vi "Magnetometer_Test_v0.vi"() -> ()   [LabVIEW 2019]
uses:
  <vilib>/DAQmx/write.llb/DAQmx Write (Analog DBL 1Chan 1Samp).vi
  <vilib>/DAQmx/read.llb/DAQmx Read (Analog 1D Wfm NChan NSamp).vi
  <extravilib>/ChannelInstances/Tag-c(bool,i32,str)/Read With Abort.vi
  <extravilib>/ChannelInstances/Tag-a[.](wfm(dbl))/Read With Abort.vi
  <extravilib>/ChannelInstances/Tag-bool/Read With Abort.vi
  <extravilib>/ChannelInstances/Tag-bool/Write With Abort.vi
  <extravilib>/ChannelInstances/Tag-c(bool,i32,str)/Write With Abort.vi
  <extravilib>/ChannelInstances/Tag-a[.](wfm(dbl))/Write With Abort.vi
  <vilib>/DAQmx/create/channels.llb/DAQmx Create Channel (AI-Voltage-Basic).vi
  <vilib>/DAQmx/configure/timing.llb/DAQmx Timing (Sample Clock).vi
  <vilib>/Utility/file.llb/Write Delimited Spreadsheet (string).vi
  <vilib>/DAQmx/create/channels.llb/DAQmx Create Channel (AO-Voltage-Basic).vi
  <extravilib>/ChannelInstances/Tag-bool/Instantiate.vi
  <extravilib>/ChannelInstances/Tag-bool/EndpointRead.vi
  <vilib>/DAQmx/miscellaneous.llb/DAQmx Fill In Error Info.vi
  <extravilib>/ChannelInstances/Tag-bool/Endpoint.vi
  <extravilib>/ChannelInstances/Tag-a[.](wfm(dbl))/Instantiate.vi
  <extravilib>/ChannelInstances/Tag-c(bool,i32,str)/Instantiate.vi
  <extravilib>/ChannelInstances/Tag-c(bool,i32,str)/EndpointRead.vi
  <extravilib>/ChannelInstances/Tag-a[.](wfm(dbl))/EndpointRead.vi
  <vilib>/imath/engines/lvmath2/RunTimeEngine/Managers/WorkSpace/UID Generator.vi
  <vilib>/imath/engines/lvmath2/RunTimeEngine/RunTimeType/NIMS_RunTimeType_From StrictType (excl LVString).vi
  <instcachedir>/0/NIMS_RunTimeType_From StrictType (excl LVString)_D8AFBA86A94845AAA577C895450664BD.lvgen/NIMS_RunTimeType_From StrictType (excl LVString)_D8AFBA86A94845AAA577C895450664BD_000.vi
  <vilib>/imath/engines/lvmath2/RunTimeEngine/LocalVariableDefStatement/MC_LocalVariableDefStatement_Display.vi
  <vilib>/imath/engines/lvmath2/RunTimeEngine/ArithmeticOperatorToken/NIMS_ArithmeticOperator_power(S).vi
  <instcachedir>/0/NIMS_ArithmeticOperator_power(S)_F1497A2DE3CE4E82B2C3646D59904248.lvgen/NIMS_ArithmeticOperator_power(S)_F1497A2DE3CE4E82B2C3646D59904248_010.vi
  <vilib>/imathl/engines/lvmath/Functions/Error Handling/Create Error.vi
  <vilib>/imath/engines/lvmath2/RunTimeEngine/Managers/SymbolTable/Clear UID.vi
  <vilib>/imath/engines/lvmath2/RunTimeEngine/NodeEndStatement/NIMS_NodeEndStatement_Output.vi
  <instcachedir>/0/NIMS_NodeEndStatement_Output_53EC0D466D134D7ABD903AC30B43404B.lvgen/NIMS_NodeEndStatement_Output_53EC0D466D134D7ABD903AC30B43404B_009.vi
  <vilib>/imath/engines/lvmath2/RunTimeEngine/ErrorHandling/NIMS_Finalize Error.vi
  <extravilib>/ChannelInstances/Tag-a[.](wfm(dbl))/Endpoint.vi
  <extravilib>/ChannelInstances/Tag-c(bool,i32,str)/Endpoint.vi
  <vilib>/DAQmx/write.llb/DAQmx Write (Analog 1D DBL NChan 1Samp).vi
  <resource>/objmgr/daqmx.rc
  <extravilib>/ChannelInstances/Tag-bool.lvlib
  <extravilib>/ChannelInstances/Tag-c(bool,i32,str).lvlib
  <extravilib>/ChannelInstances/Tag-a[.](wfm(dbl)).lvlib
  <vilib>/imath/engines/lvmath2/RunTimeEngine/Managers/SymbolTable/NIMS_WorkSpace.lvlib
panel:
  in  "Data Record Work Rate (ms)":u16(ring)=100 items=["100"=100, "250"=250, "500"=500, "1000"=1000, "2500"=2500, "5000"=5000, ""=0]
  out "Magnetic Field Indicator":dbl
  out "Magnetic Field":dbl(graph)
  out "Temperature (VDC)":dbl
  out "Temperature (Celsius)":dbl
  out "Temperature":dbl(slide) scale=-40.0..160.0
  in  "Temperature \nMeasurement On/Off":bool=TRUE
  out "TCP Connection":bool
  in  "Reset":bool
  out "Output 2 Current In Range?":bool
  out "Output 1 Current In Range?":bool
  out "Output 2 Input Current":string
  out "Output 1 Measured Current":string
  out "Output 2 Input Voltage":string
  out "Output 2 Measured Current":string
  out "Output 2 Measured Voltage":string
  out "Output 1 Input Current":string
  out "Output 1 Input Voltage":string
  out "Output 1 Measured Voltage":string
  in  "Output On/Off":bool
  out "Iteration of PS Controller":dbl
  out "MtM Z-Axis Output Voltage":string
  out "MtM Y-Axis Output Voltage":string
  in  "Data History Work Rate (ms)":u16(ring)=1000 items=["100"=100, "250"=250, "500"=500, "1000"=1000, "2500"=2500, "5000"=5000, ""=0]
  out "MtM X-Axis Output Voltage":string
  in  "Simulation On/Off":bool
  in  "Sample Clock Source":tag="OnboardClock"
  out "MtM Z-Axis Output Voltage":waveform(dbl)(graph)
  out "MtM Y-Axis Output Voltage":waveform(dbl)(graph)
  out "MtM X-Axis Output Voltage":waveform(dbl)(graph)
  in  "MtM Z-Axis Input Voltage":dbl
  in  "MtM Y-Axis Input Voltage":dbl
  in  "MtM X-Axis Input Voltage":dbl
  in  "Acquire Buffer Size":i32=1024
  in  "Sample Rate":dbl=1000.0 format="%0.2f"
  out "DAQmx Read Rate":dbl
  in  "Number of Samples":i32=100
  out "While loop duration (ms)":u32
  in  "Stop":bool
  # "Sensor Output"
  # "Data Acqusition Timing and\nBuffer Settings"
  # "Temperature Output"
  # "Acquire Data History"
  # "Magnetic Field Output"
  # "Power Supply Control and Status"
  # "Simulation of Analogue Voltage Generation"
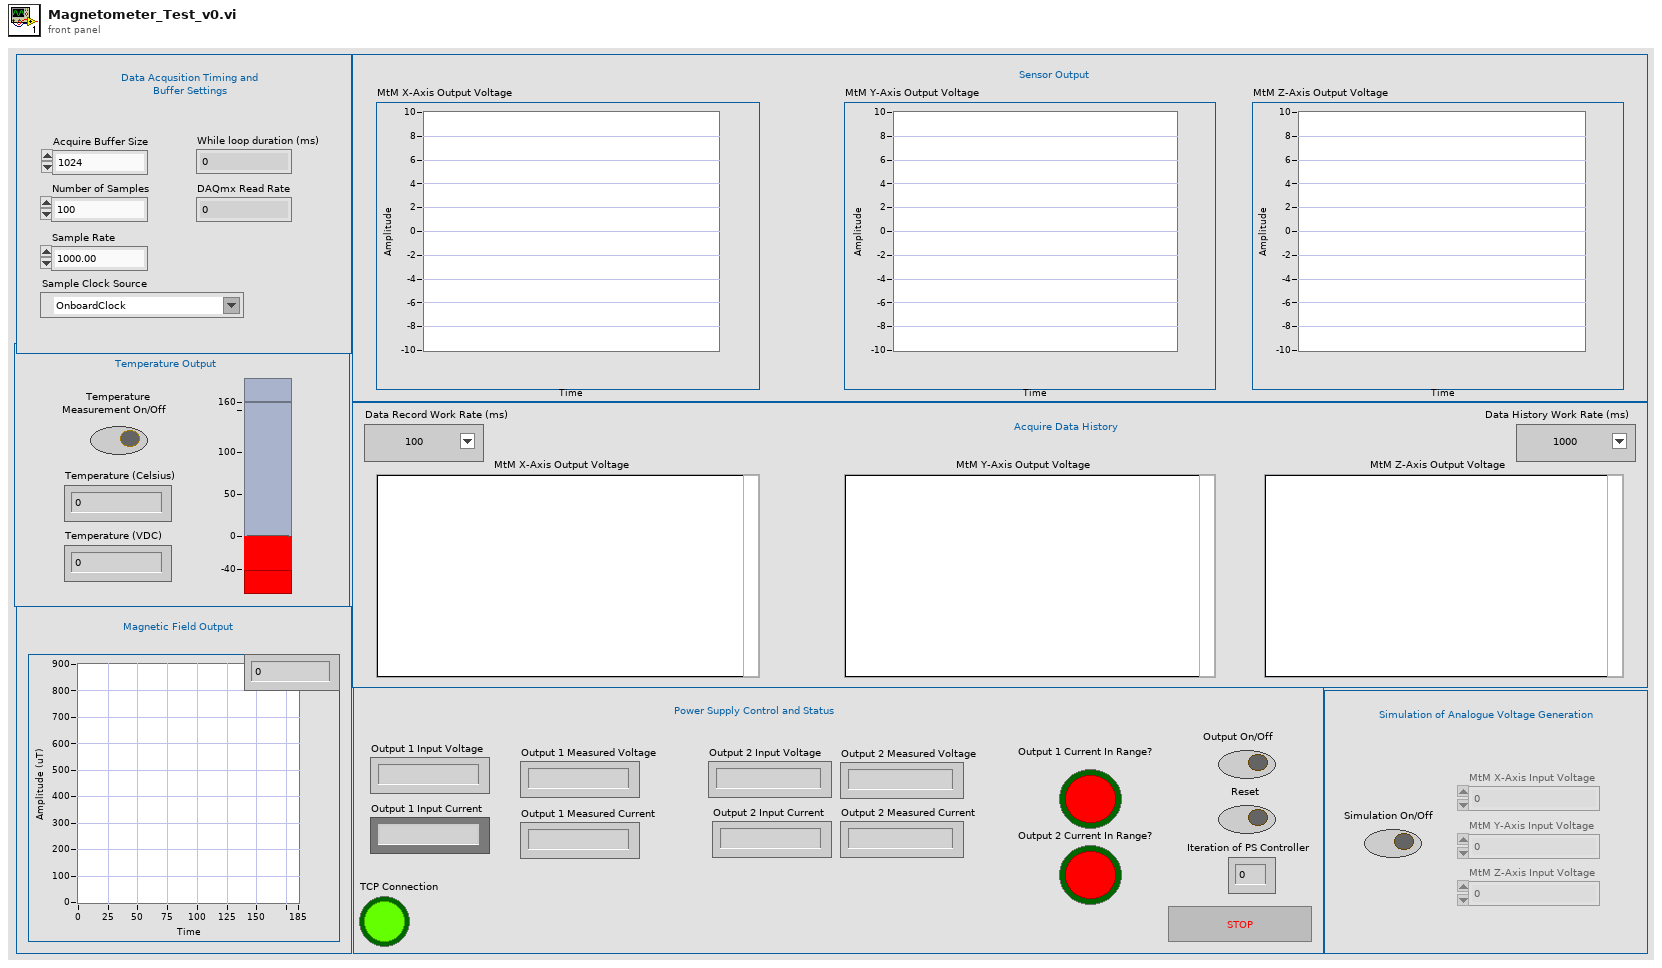
[diagram p1: front panel]
types:
  T1 = typedef "Tag-bool.lvlib/))Channel.ctl" = refnum<queue>
  T2 = typedef "Tag-a[.](wfm(dbl)).lvlib/))Channel.ctl" = refnum<queue>
  T3 = typedef "Tag-c(bool,i32,str).lvlib/))Channel.ctl" = refnum<queue>
  T4 = enum8{"Enabled", "Disabled", "Disabled and Grayed Out"}
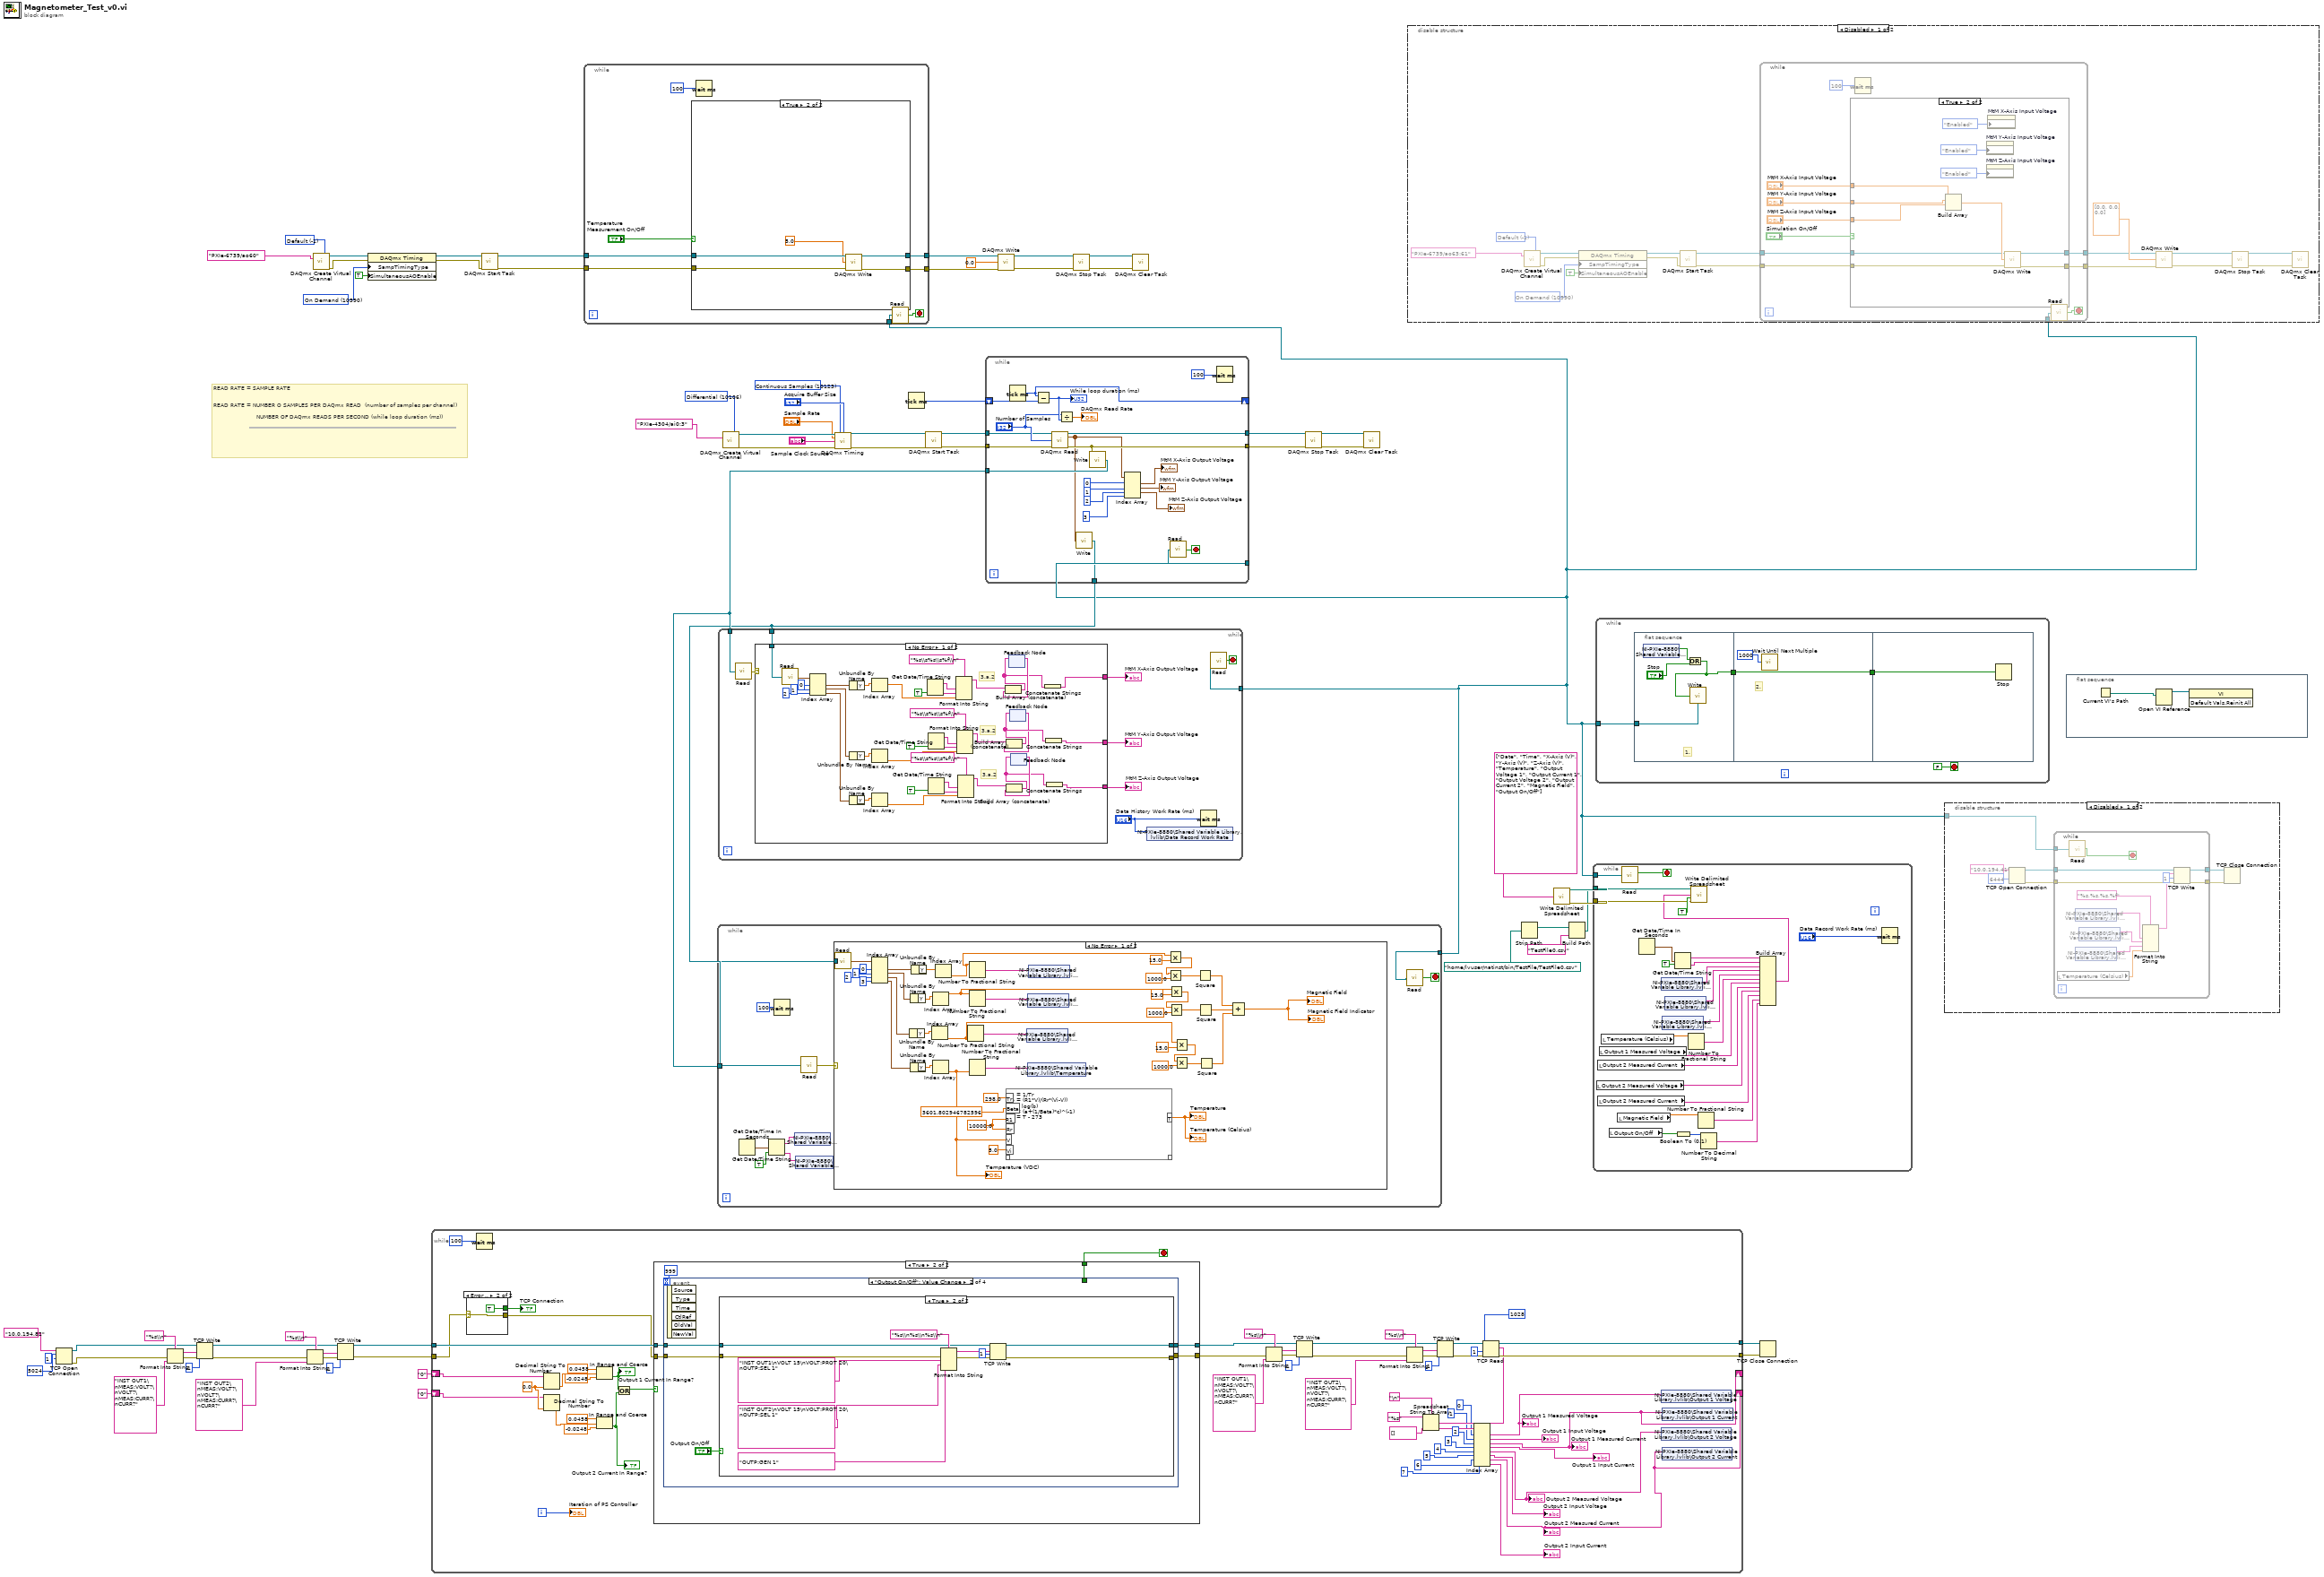
[diagram p0: block diagram]
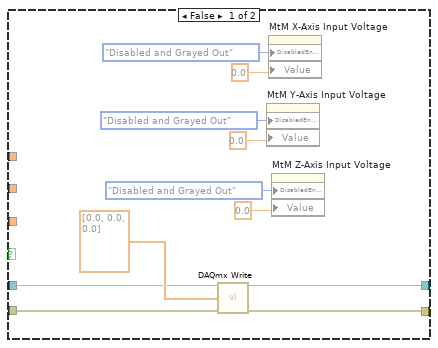
[diagram p4: hidden frame]
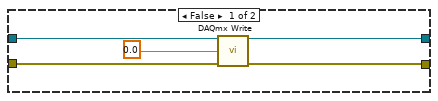
[diagram p6: hidden frame]
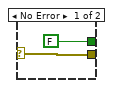
[diagram p7: hidden frame]
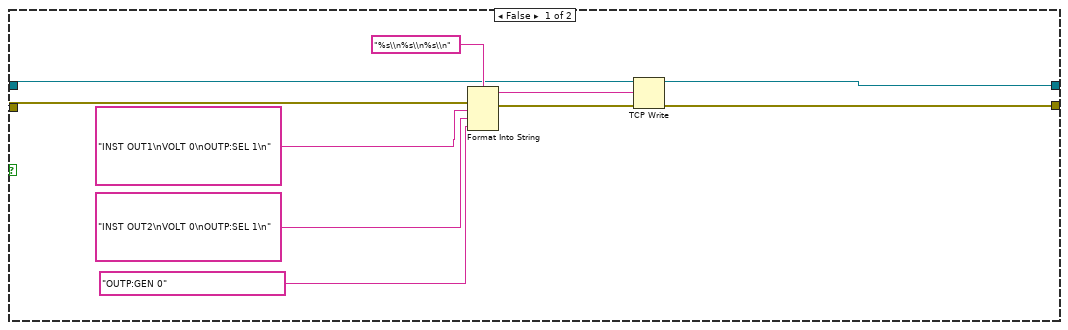
[diagram p8: hidden frame]
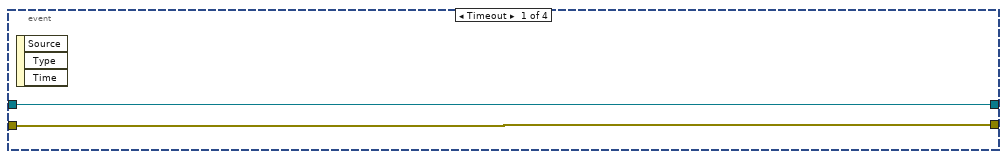
[diagram p9: hidden frame]
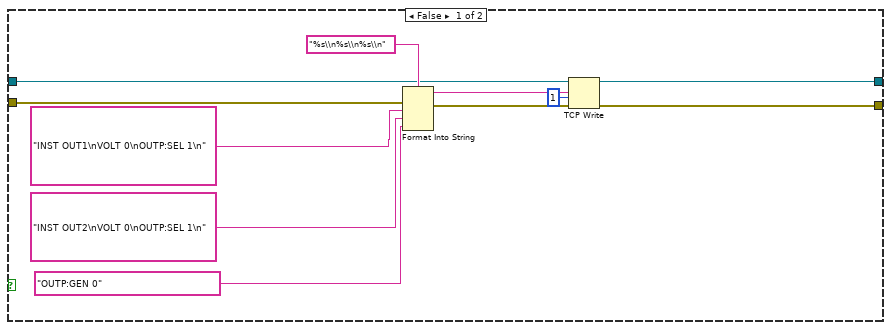
[diagram p10: hidden frame]
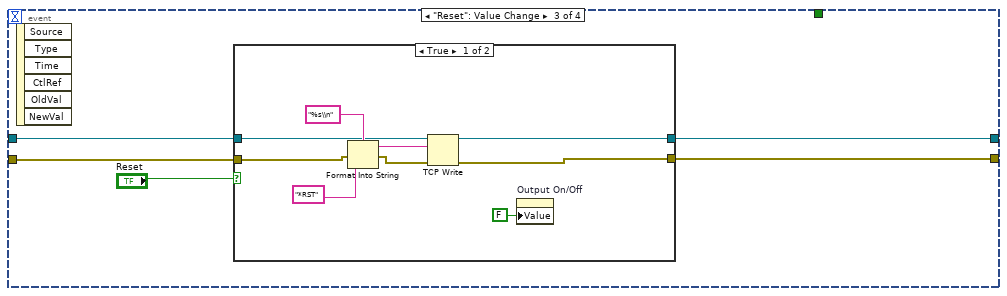
[diagram p11: hidden frame]
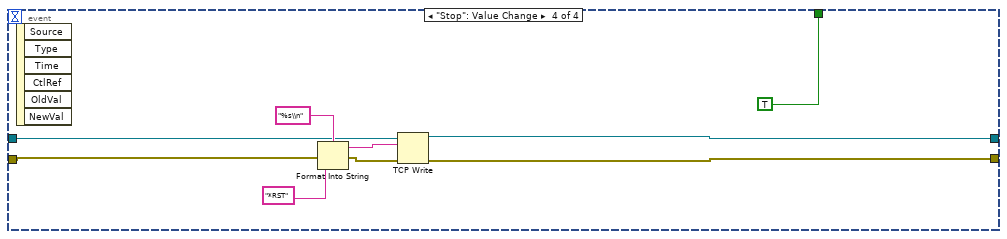
[diagram p13: hidden frame]
diagram:
  w17 = 10390 items=["Sample Clock"=10388, "Burst Handshake"=12548, "Handshake"=10389, "Implicit"=10451, "On Demand"=10390, "Change Detection"=12504, "Pipelined Sample Clock"=14668] ("SampTimingType")
  w22 = -1 items=["Default"=-1, "RSE"=10083, "Differential"=10106, "Pseudodifferential"=12529] ("output terminal configuration")
  w54 = 10123 items=["Finite Samples"=10178, "Continuous Samples"=10123, "Hardware Timed Single Point"=12522] ("sample mode")
  w67 = 10106 items=["Default"=-1, "RSE"=10083, "NRSE"=10078, "Differential"=10106, "Pseudodifferential"=12529] ("input terminal configuration")
  # "READ RATE = SAMPLE RATE\n\n\nREAD RATE = NUMBER O SAMPLES PER DAQmx READ  (number of samples per channel)\n\n                        NUMBER OF DAQmx READS PER SECOND (while loop duration (ms))"
  n1 = TCP Open Connection(address="10.0.194.82", remote port or service name=u16 5024, timeout ms (60000)=1) -> (connection ID=w25:refnum<k5>, error out=w26:errorcluster)  [unwired: 2 in]
  n2 = Format Into String(format string="%s\\n", error in=w26, "INST OUT1\nMEAS:VOLT?\nVOLT?\nMEAS:CURR?\nCURR?") -> (resulting string=w32:string, error out=w34:errorcluster)  [unwired: 1 in]
  n3 = TCP Write(connection ID=w25, data in=w32, error in (no error)=w34, 9:1 ("timeout ms (25000)")) -> (connection ID out=w30:refnum<k5>, error out=w29:errorcluster)  [unwired: 1 out]
  n4 = Format Into String(format string="%s\\n", error in=w29, "INST OUT2\nMEAS:VOLT?\nVOLT?\nMEAS:CURR?\nCURR?") -> (resulting string=w36:string, error out=w38:errorcluster)  [unwired: 1 in]
  n5 = call-poly <vilib>:"DAQmx Create Virtual Channel.vi"("output terminal configuration"=w22, "physical channels"=tag "PXIe-6739/ao60") -> ("task out"=w19:refnum<k21>, "error out"=w18:errorcluster)  [unwired: 12 in]
  n6 = TCP Write(connection ID=w30, data in=w36, error in (no error)=w38, 9:1 ("timeout ms (25000)")) -> (connection ID out=w28:refnum<k5>, error out=w27:errorcluster)  [unwired: 1 out]
  n7 = property class="DAQmx Timing"(reference=w19, error in=w18, "SampTimingType"=w17, "SimultaneousAOEnable"=TRUE) -> (reference out=w21:refnum<k21>, error out=w20:errorcluster)
  n8 = while {
    tunnel: w28 -> [w124]
    tunnel: w27 -> [w74]
    tunnel: [w127] -> w48
    tunnel: [w126] -> w47
    shift-right: [w71] -> _
    shift-left: "0" -> [w70]
    shift-right: [w69] -> _
    shift-left: "0" -> [w68]
    i -> [w125]
    stop <- w123 stop-if-true
    w122 = 0.0
    n9 = case shown="Error .." w74 {
      selector: w74 -> [w128 w130]
      tunnel: [FALSE ("TCP Connection") TRUE ("TCP Connection")] -> w73
      tunnel: [w128 w130] -> w72
      frame No Error {
      }
      frame Error {
      }
    }
    "TCP Connection" <- w73
    n10 = Wait (ms)(milliseconds to wait=u32 100 ("millisecond multiple")) -> ()  [unwired: 1 out]
    n11 = Decimal String To Number(string=w70, default (0L)=w122) -> (number=w116:dbl)  [unwired: 1 in, 1 out]
    n12 = Decimal String To Number(string=w68, default (0L)=w122) -> (number=w115:dbl)  [unwired: 1 in, 1 out]
    n13 = In Range and Coerce(upper limit=0.0458 ("y"), x=w115, lower limit=-0.0248 ("y")) -> (In Range?=w101:bool)  [unwired: 1 out]
    "Output 2 Current In Range?" <- w101
    n14 = In Range and Coerce(upper limit=0.0458 ("y"), x=w116, lower limit=-0.0248 ("y")) -> (In Range?=w114:bool)  [unwired: 1 out]
    "Output 1 Current In Range?" <- w114
    n15 = Or(x=w114, y=w101) -> (x .or. y?=w102:bool)
    n16 = case shown="True" w102 {
      tunnel: w124 -> [w135 w147]
      tunnel: w72 -> [w134 w146]
      tunnel: [_ w145] -> w123
      tunnel: [w132 w143] -> w77
      tunnel: [w133 w142] -> w76
      frame False {
        n17 = Format Into String(format string="%s\\n%s\\n%s\\n", error in=w134, "INST OUT1\nVOLT 0\nOUTP:SEL 1\n", "INST OUT2\nVOLT 0\nOUTP:SEL 1\n", "OUTP:GEN 0") -> (resulting string=w140:string, error out=w141:errorcluster)  [unwired: 1 in]
        n18 = TCP Write(connection ID=w135, data in=w140, error in (no error)=w141) -> (connection ID out=w132:refnum<k5>, error out=w133:errorcluster)  [unwired: 1 in, 1 out]
      }
      frame True {
        n19 = event shown="[1] \"Output On/Off\": Value Change" {
          selector: _ -> [_ _ _ _]
          dyn-events: _ -> [_ _ _ _]
          timeout: 999 -> [_ _ _ _]
          tunnel: [w148 w154 w179 w194] -> w143
          tunnel: [w149 w152 w178 w193] -> w142
          tunnel: w147 -> [w148 w151 w181 w196]
          tunnel: w146 -> [w149 w150 w180 w197]
          tunnel: [_ _ _ TRUE] -> w145
          event Timeout {
            n20 = event-data() -> ()  [unwired: 1 in, 3 out]
          }
          event "Output On/Off": Value Change {
            n21 = event-data() -> ()  [unwired: 1 in, 6 out]
            n22 = case shown="True" "Output On/Off" {
              tunnel: [w157 w171] -> w154
              tunnel: [w156 w170] -> w152
              tunnel: w151 -> [w159 w173]
              tunnel: w150 -> [w158 w172]
              frame False {
                n23 = Format Into String(format string="%s\\n%s\\n%s\\n", error in=w158, "INST OUT1\nVOLT 0\nOUTP:SEL 1\n", "INST OUT2\nVOLT 0\nOUTP:SEL 1\n", "OUTP:GEN 0") -> (resulting string=w164:string, error out=w165:errorcluster)  [unwired: 1 in]
                n24 = TCP Write(connection ID=w159, data in=w164, error in (no error)=w165, 9:1 ("timeout ms (25000)")) -> (connection ID out=w157:refnum<k5>, error out=w156:errorcluster)  [unwired: 1 out]
              }
              frame True {
                n25 = Format Into String(format string="%s\\n%s\\n%s\\n", error in=w172, "INST OUT1\nVOLT 15\nVOLT:PROT 20\nOUTP:SEL 1", "INST OUT2\nVOLT 15\nVOLT:PROT 20\nOUTP:SEL 1", "OUTP:GEN 1") -> (resulting string=w174:string, error out=w176:errorcluster)  [unwired: 1 in]
                n26 = TCP Write(connection ID=w173, data in=w174, error in (no error)=w176, 9:1 ("timeout ms (25000)")) -> (connection ID out=w171:refnum<k5>, error out=w170:errorcluster)  [unwired: 1 out]
              }
            }
          }
          event "Reset": Value Change {
            n27 = event-data() -> ()  [unwired: 1 in, 6 out]
            n28 = case shown="True" "Reset" {
              tunnel: [w184 w192] -> w179
              tunnel: [w183 w191] -> w178
              tunnel: w181 -> [w185 w192]
              tunnel: w180 -> [w186 w191]
              frame True {
                n29 = Format Into String(format string="%s\\n", error in=w186, "*RST" ("data in")) -> (resulting string=w188:string, error out=w187:errorcluster)  [unwired: 1 in]
                n30 = TCP Write(connection ID=w185, data in=w188, error in (no error)=w187) -> (connection ID out=w184:refnum<k5>, error out=w183:errorcluster)  [unwired: 1 in, 1 out]
                n31 = property on="Output On/Off" class="Bool (strict)"("Value"=FALSE ("Output On/Off")) -> ()  [unwired: 2 in, 2 out]
              }
              frame False {
              }
            }
          }
          event "Stop": Value Change {
            n32 = event-data() -> ()  [unwired: 1 in, 6 out]
            n33 = Format Into String(format string="%s\\n", error in=w197, "*RST" ("data in")) -> (resulting string=w199:string, error out=w198:errorcluster)  [unwired: 1 in]
            n34 = TCP Write(connection ID=w196, data in=w199, error in (no error)=w198) -> (connection ID out=w194:refnum<k5>, error out=w193:errorcluster)  [unwired: 1 in, 1 out]
          }
        }
      }
    }
    n35 = Format Into String(format string="%s\\n", error in=w76, "INST OUT1\nMEAS:VOLT?\nVOLT?\nMEAS:CURR?\nCURR?") -> (resulting string=w81:string, error out=w83:errorcluster)  [unwired: 1 in]
    n36 = TCP Write(connection ID=w77, data in=w81, error in (no error)=w83, 9:1 ("timeout ms (25000)")) -> (connection ID out=w79:refnum<k5>, error out=w78:errorcluster)  [unwired: 1 out]
    n37 = Format Into String(format string="%s\\n", error in=w78, "INST OUT2\nMEAS:VOLT?\nVOLT?\nMEAS:CURR?\nCURR?") -> (resulting string=w106:string, error out=w108:errorcluster)  [unwired: 1 in]
    n38 = TCP Write(connection ID=w79, data in=w106, error in (no error)=w108, 9:1 ("timeout ms (25000)")) -> (connection ID out=w105:refnum<k5>, error out=w104:errorcluster)  [unwired: 1 out]
    n39 = TCP Read(connection ID=w105, bytes to read=1028, error in (no error)=w104, 9:1 ("timeout ms (25000)")) -> (connection ID out=w127:refnum<k5>, data out=w109:string, error out=w126:errorcluster)  [unwired: 1 in]
    n40 = Spreadsheet String To Array(delimiter (Tab)="\n", format string="%s", spreadsheet string=w109, array type (2D Dbl)=string[] []) -> (array=w111:string[])
    n41 = Index Array(array=w111, index #1=0 ("index"), index #2=1 ("index"), index #3=2 ("index"), index #4=3 ("index"), index #5=4 ("index"), index #6=5 ("index"), index #7=6 ("index"), index #8=7 ("index")) -> (element #1=w100:string, element #2=→"Output 1 Input Voltage":string, element #3=w71:string, element #4=→"Output 1 Input Current":string, element #5=w96:string, element #6=→"Output 2 Input Voltage":string, element #7=w69:string, element #8=→"Output 2 Input Current":string)
    "Output 1 Measured Voltage" <- w100
    "Output 2 Measured Voltage" <- w96
    "Output 2 Measured Current" <- w69
    "Output 1 Measured Current" <- w71
    n42 = shared-variable "NI-PXIe-8880\\Shared Variable Library.lvlib\\Output 1 Voltage"(w100) -> ()  [unwired: 1 in, 1 out]
    n43 = shared-variable "NI-PXIe-8880\\Shared Variable Library.lvlib\\Output 2 Voltage"(w96) -> ()  [unwired: 1 in, 1 out]
    n44 = shared-variable "NI-PXIe-8880\\Shared Variable Library.lvlib\\Output 2 Current"(w69) -> ()  [unwired: 1 in, 1 out]
    n45 = shared-variable "NI-PXIe-8880\\Shared Variable Library.lvlib\\Output 1 Current"(w71) -> ()  [unwired: 1 in, 1 out]
    "Iteration of PS Controller" <- w125
  }
  n46 = call <vilib>:"DAQmx Start Task.vi"("task/channels in"=w21, "error in"=w20) -> ("task out"=w14:refnum<k21>, "error out"=w13:errorcluster)  [unwired: 12 in]
  n47 = call-poly <vilib>:"DAQmx Create Virtual Channel.vi"("input terminal configuration"=w67, "physical channels"=tag "PXIe-4304/ai0:3") -> ("task out"=w59:refnum<k21>, "error out"=w58:errorcluster)  [unwired: 12 in]
  n48 = call-poly <vilib>:"DAQmx Timing.vi"("task/channels in"=w59, "sample mode"=w54, "samples per channel"="Acquire Buffer Size", "rate"="Sample Rate", "source"="Sample Clock Source", "error in"=w58) -> ("task out"=w56:refnum<k21>, "error out"=w57:errorcluster)  [unwired: 8 in]
  n49 = Tick Count (ms)() -> (millisecond timer value=w60:u32)
  n50 = call <vilib>:"DAQmx Start Task.vi"("task/channels in"=w56, "error in"=w57) -> ("task out"=w65:refnum<k21>, "error out"=w66:errorcluster)  [unwired: 12 in]
  n51 = Strip Path(path=path "/home/lvuser/natinst/bin/TestFile/TestFile0.csv") -> (stripped path=w46:path)  [unwired: 1 out]
  n52 = Build Path(base path=w46, name or relative path="TestFile0.csv") -> (appended path=w41:path)
  n53 = call-poly <vilib>:"Write Delimited Spreadsheet.vi"("file path (dialog if empty)"=w41, "1D data"=string[] ["Date", "Time", "X-Axis (V)", "Y-Axis (V)", "Z-Axis (V)", "Temperature", "Output Voltage 1", "Output Current 1", "Output Voltage 2", "Output Current 2", "Magnetic Field", "Output On/Off"]) -> ("new file path (Not A Path if cancelled)"=w43:path, "error out"=w42:errorcluster)  [unwired: 12 in]
  n54 = while {
    tunnel: [w203] -> w1
    stop <- FALSE stop-if-true
    n55 = flat-sequence {
      tunnel: [w206] -> w204
      tunnel: [w209] -> w203
      tunnel: w204 -> [w211]
      tunnel: [w211] -> w202
      tunnel: w202 -> [w212]
      frame #0 {
        # "1."
        n56 = shared-variable "NI-PXIe-8880\\Shared Variable Library.lvlib\\Stop"() -> (w207:bool)  [unwired: 1 in, 1 out]
        n57 = Or(x=w207, y="Stop") -> (x .or. y?=w206:bool)
        n58 = call <extravilib>:"Write.vi"("element"=w206) -> ("channel"=w209:T1)  [unwired: 1 out]
      }
      frame #1 {
        # "2."
        n59 = call "Wait Until Next Multiple"("Count(mSec)"=u32 1000) -> ()  [unwired: 1 out]
      }
      frame #2 {
        n60 = Stop(stop? (T)=w212) -> ()
      }
    }
  }
  n61 = while {
    tunnel: w14 -> [w220]
    tunnel: w13 -> [w219]
    tunnel: [w218] -> w8
    tunnel: [w217] -> w7
    tunnel: w1 -> [w216]
    stop <- w215 stop-if-true
    n62 = case shown="True" "Temperature \nMeasurement On/Off" {
      tunnel: w220 -> [w223 w230]
      tunnel: w219 -> [w222 w229]
      tunnel: [w225 w228] -> w218
      tunnel: [w224 w227] -> w217
      frame False {
        n63 = call-poly <vilib>:"DAQmx Write.vi"("task/channels in"=w223, "data"=0.0 ("Waveform"), "error in"=w222) -> ("task out"=w225:refnum<k21>, "error out"=w224:errorcluster)  [unwired: 10 in, 1 out]
      }
      frame True {
        n64 = call-poly <vilib>:"DAQmx Write.vi"("task/channels in"=w230, "data"=5.0 ("MtM X-Axis Input Voltage 2"), "error in"=w229) -> ("task out"=w228:refnum<k21>, "error out"=w227:errorcluster)  [unwired: 10 in, 1 out]
      }
    }
    n65 = Wait (ms)(milliseconds to wait=u32 100) -> ()  [unwired: 1 out]
    n66 = call <extravilib>:"Read.vi"("channel"=w216) -> ("element"=w215:bool)  [unwired: 1 in, 1 out]
  }
  n67 = while {
    shift-right: [w247] -> _
    shift-left: w60 -> [w250]
    tunnel: w65 -> [w244]
    tunnel: [w252] -> w64
    tunnel: w66 -> [w243]
    tunnel: [w251] -> w63
    tunnel: [w237] -> w5
    tunnel: [w235] -> w4
    tunnel: w1 -> [w234]
    stop <- w233 stop-if-true
    n68 = Tick Count (ms)() -> (millisecond timer value=w247:u32)
    n69 = Subtract(x=w247, y=w250) -> (x-y=w246:u32)
    "While loop duration (ms)" <- w246
    n70 = call-poly <vilib>:"DAQmx Read.vi"("task/channels in"=w244, "number of samples per channel"="Number of Samples", "error in"=w243) -> ("task out"=w252:refnum<k21>, "data"=w236:waveform(dbl)[], "error out"=w251:errorcluster)  [unwired: 10 in]
    n71 = Divide(x="Number of Samples", y=w246) -> (x/y=→"DAQmx Read Rate":dbl)
    n72 = call <extravilib>:"Write.vi"("element"=w236) -> ("channel"=w235:T2)  [unwired: 1 out]
    n73 = call <extravilib>:"Write.vi"("element"=w251) -> ("channel"=w237:T3)  [unwired: 1 out]
    n74 = Index Array(array=w236, index #1=0 ("index"), index #2=1 ("index"), index #3=2 ("index"), index #4=3 ("index")) -> (element #1=→"MtM X-Axis Output Voltage":waveform(dbl), element #2=→"MtM Y-Axis Output Voltage":waveform(dbl), element #3=→"MtM Z-Axis Output Voltage":waveform(dbl))  [unwired: 1 out]
    n75 = call <extravilib>:"Read.vi"("channel"=w234) -> ("element"=w233:bool)  [unwired: 1 in, 1 out]
    n76 = Wait (ms)(milliseconds to wait=u32 100) -> ()  [unwired: 1 out]
  }
  n77 = while {
    tunnel: w1 -> [w261]
    tunnel: w5 -> [w259]
    tunnel: w4 -> [w258]
    stop <- w262 stop-if-true
    n78 = Get Date/Time In Seconds() -> (seconds since 1Jan1904=w255:timestamp)
    n79 = Get Date/Time String(seconds (now)=w255, want seconds? (F)=TRUE) -> (date string=w256:string, time string=w257:string)  [unwired: 1 in]
    n80 = Wait (ms)(milliseconds to wait=u32 100) -> ()  [unwired: 1 out]
    n81 = shared-variable "NI-PXIe-8880\\Shared Variable Library.lvlib\\Date"(w256) -> ()  [unwired: 1 in, 1 out]
    n82 = shared-variable "NI-PXIe-8880\\Shared Variable Library.lvlib\\Time"(w257) -> ()  [unwired: 1 in, 1 out]
    n83 = call <extravilib>:"Read.vi"("channel"=w259) -> ("element"=w260:errorcluster)  [unwired: 1 in, 1 out]
    n84 = case shown="No Error" w260 {
      tunnel: w258 -> [w274 _]
      frame No Error {
        w295 = 10000.0 ("R1")
        n85 = call <extravilib>:"Read.vi"("channel"=w274) -> ("element"=w273:waveform(dbl)[])  [unwired: 1 in, 1 out]
        n86 = Index Array(array=w273, index #1=0 ("index"), index #2=1 ("index"), index #3=2 ("index"), index #4=3 ("index")) -> (element #1=w272:waveform(dbl), element #2=w271:waveform(dbl), element #3=w266:waveform(dbl), element #4=w269:waveform(dbl))
        n87 = Unbundle By Name(w266) -> ("Y"=w267:dbl[])
        n88 = Unbundle By Name(w271) -> ("Y"=w270:dbl[])
        n89 = Unbundle By Name(w269) -> ("Y"=w268:dbl[])
        n90 = Unbundle By Name(w272) -> ("Y"=w265:dbl[])
        n91 = Index Array(array=w267) -> (element=w275:dbl)  [unwired: 1 in]
        n92 = Index Array(array=w270) -> (element=w276:dbl)  [unwired: 1 in]
        n93 = Index Array(array=w268) -> (element=w292:dbl)  [unwired: 1 in]
        "Temperature (VDC)" <- w292
        n94 = Index Array(array=w265) -> (element=w264:dbl)  [unwired: 1 in]
        n95 = Number To Fractional String(number=w275) -> (F-format string=w299:string)  [unwired: 3 in]
        n96 = Number To Fractional String(number=w276) -> (F-format string=w300:string)  [unwired: 3 in]
        n97 = Number To Fractional String(number=w292) -> (F-format string=w298:string)  [unwired: 3 in]
        n98 = Number To Fractional String(number=w264) -> (F-format string=w301:string)  [unwired: 3 in]
        n99 = mathscript code="a = 1/Tr\nb = (R1*V)/(Rr*(Vi-V))\nc = log(b)\nT = (a+(1/Beta)*c)^(-1)\nT = T - 273"("Tr"=298.0, "Beta"=3601.802946782596, "R1"=w295, "Rr"=w295, "V"=w292, "Vi"=5.0) -> ("T"=→"Temperature" →"Temperature (Celsius)":cdb)  [unwired: 1 in, 1 out]
        n100 = shared-variable "NI-PXIe-8880\\Shared Variable Library.lvlib\\Z-Axis"(w299) -> ()  [unwired: 1 in, 1 out]
        n101 = shared-variable "NI-PXIe-8880\\Shared Variable Library.lvlib\\Y-Axis"(w300) -> ()  [unwired: 1 in, 1 out]
        n102 = shared-variable "NI-PXIe-8880\\Shared Variable Library.lvlib\\Temperature"(w298) -> ()  [unwired: 1 in, 1 out]
        n103 = shared-variable "NI-PXIe-8880\\Shared Variable Library.lvlib\\X-Axis"(w301) -> ()  [unwired: 1 in, 1 out]
        n104 = Multiply(x=w264, y=15.0) -> (x*y=w290:dbl)
        n105 = Multiply(x=w290, y=1000.0) -> (x*y=w286:dbl)
        n106 = Multiply(x=w276, y=15.0) -> (x*y=w285:dbl)
        n107 = Multiply(x=w285, y=1000.0) -> (x*y=w284:dbl)
        n108 = Multiply(x=w275, y=15.0) -> (x*y=w280:dbl)
        n109 = Multiply(x=w280, y=1000.0) -> (x*y=w281:dbl)
        n110 = Square(x=w286) -> (x^2=w278:dbl)
        n111 = Square(x=w284) -> (x^2=w279:dbl)
        n112 = Square(x=w281) -> (x^2=w277:dbl)
        n113 = Compound Arithmetic op=ADD(w278, w279, w277) -> (→"Magnetic Field" →"Magnetic Field Indicator":dbl)
      }
      frame Error {
      }
    }
    n114 = call <extravilib>:"Read.vi"("channel"=w261) -> ("element"=w262:bool)  [unwired: 1 in, 1 out]
  }
  n115 = while {
    tunnel: w5 -> [w439]
    tunnel: w4 -> [w438]
    tunnel: w1 -> [w437]
    stop <- w436 stop-if-true
    n116 = call <extravilib>:"Read.vi"("channel"=w439) -> ("element"=w435:errorcluster)  [unwired: 1 in, 1 out]
    n117 = case shown="No Error" w435 {
      tunnel: w438 -> [w472 _]
      tunnel: [w465 _] -> w434
      tunnel: [w457 _] -> w433
      tunnel: [w456 _] -> w432
      frame No Error {
        # "3.a.2"
        # "3.a.2"
        # "3.a.2"
        n118 = call <extravilib>:"Read.vi"("channel"=w472) -> ("element"=w468:waveform(dbl)[])  [unwired: 1 in, 1 out]
        n119 = Index Array(array=w468, index #1=0 ("index"), index #2=1 ("index"), index #3=2 ("index")) -> (element #1=w448:waveform(dbl), element #2=w447:waveform(dbl), element #3=w446:waveform(dbl))
        n120 = Unbundle By Name(w448) -> ("Y"=w445:dbl[])
        n121 = Unbundle By Name(w447) -> ("Y"=w444:dbl[])
        n122 = Unbundle By Name(w446) -> ("Y"=w443:dbl[])
        n123 = Index Array(array=w445) -> (element=w440:dbl)  [unwired: 1 in]
        n124 = Index Array(array=w444) -> (element=w441:dbl)  [unwired: 1 in]
        n125 = Index Array(array=w443) -> (element=w442:dbl)  [unwired: 1 in]
        n126 = Get Date/Time String(want seconds? (F)=TRUE) -> (date string=w467:string, time string=w466:string)  [unwired: 2 in]
        n127 = Get Date/Time String(want seconds? (F)=TRUE) -> (date string=w463:string, time string=w464:string)  [unwired: 2 in]
        n128 = Get Date/Time String(want seconds? (F)=TRUE) -> (date string=w450:string, time string=w449:string)  [unwired: 2 in]
        n129 = Format Into String(format string="%s\\s%s\\s%f\\n", w467, w466, w440) -> (resulting string=w477:string)  [unwired: 2 in, 1 out]
        n130 = Format Into String(format string="%s\\s%s\\s%f\\n", w463, w464, w441) -> (resulting string=w459:string)  [unwired: 2 in, 1 out]
        n131 = Format Into String(format string="%s\\s%s\\s%f\\n", w450, w449, w442) -> (resulting string=w454:string)  [unwired: 2 in, 1 out]
        n132 = feedback #1() -> (w474:string[])  [unwired: 1 in]
        n133 = Build Array (concatenate)(w477, w474) -> (w473:string[])
        n134 = feedback-in #1(w473) -> ()
        n135 = feedback #2() -> (w461:string[])  [unwired: 1 in]
        n136 = Build Array (concatenate)(w459, w461) -> (w462:string[])
        n137 = feedback-in #2(w462) -> ()
        n138 = feedback #3() -> (w452:string[])  [unwired: 1 in]
        n139 = Build Array (concatenate)(w454, w452) -> (w451:string[])
        n140 = feedback-in #3(w451) -> ()
        n141 = Concatenate Strings(w473) -> (w465:string)
        n142 = Concatenate Strings(w462) -> (w457:string)
        n143 = Concatenate Strings(w451) -> (w456:string)
      }
      frame Error {
      }
    }
    "MtM X-Axis Output Voltage" <- w434
    "MtM Y-Axis Output Voltage" <- w433
    "MtM Z-Axis Output Voltage" <- w432
    n144 = shared-variable "NI-PXIe-8880\\Shared Variable Library.lvlib\\Data Record Work Rate"("Data History Work Rate (ms)") -> ()  [unwired: 1 in, 1 out]
    n145 = Wait (ms)(milliseconds to wait="Data History Work Rate (ms)") -> ()  [unwired: 1 out]
    n146 = call <extravilib>:"Read.vi"("channel"=w437) -> ("element"=w436:bool)  [unwired: 1 in, 1 out]
  }
  n147 = call-poly <vilib>:"DAQmx Write.vi"("task/channels in"=w8, "data"=0.0 ("Waveform"), "error in"=w7) -> ("task out"=w10:refnum<k21>, "error out"=w9:errorcluster)  [unwired: 10 in, 1 out]
  n148 = call <vilib>:"DAQmx Stop Task.vi"("task/channels in"=w10, "error in"=w9) -> ("task out"=w12:refnum<k21>, "error out"=w11:errorcluster)  [unwired: 12 in]
  n149 = call <vilib>:"DAQmx Clear Task.vi"("task in"=w12, "error in"=w11) -> ()  [unwired: 13 in, 1 out]
  n150 = call <vilib>:"DAQmx Stop Task.vi"("task/channels in"=w64, "error in"=w63) -> ("task out"=w61:refnum<k21>, "error out"=w62:errorcluster)  [unwired: 12 in]
  n151 = call <vilib>:"DAQmx Clear Task.vi"("task in"=w61, "error in"=w62) -> ()  [unwired: 13 in, 1 out]
  n152 = disable-structure shown="Disabled" {
    disable-tunnel: w1 -> [w478 _]
    frame Disabled {
      w490 = 10390 items=["Sample Clock"=10388, "Burst Handshake"=12548, "Handshake"=10389, "Implicit"=10451, "On Demand"=10390, "Change Detection"=12504, "Pipelined Sample Clock"=14668] ("SampTimingType")
      w495 = -1 items=["Default"=-1, "RSE"=10083, "Differential"=10106, "Pseudodifferential"=12529] ("output terminal configuration")
      n153 = call-poly <vilib>:"DAQmx Create Virtual Channel.vi"("output terminal configuration"=w495, "physical channels"=tag "PXIe-6739/ao63:61") -> ("task out"=w492:refnum<k21>, "error out"=w491:errorcluster)  [unwired: 12 in]
      n154 = property class="DAQmx Timing"(reference=w492, error in=w491, "SampTimingType"=w490, "SimultaneousAOEnable"=TRUE) -> (reference out=w494:refnum<k21>, error out=w493:errorcluster)
      n155 = call <vilib>:"DAQmx Start Task.vi"("task/channels in"=w494, "error in"=w493) -> ("task out"=w487:refnum<k21>, "error out"=w486:errorcluster)  [unwired: 12 in]
      n156 = while {
        tunnel: w487 -> [w506]
        tunnel: w486 -> [w505]
        tunnel: [w504] -> w480
        tunnel: [w503] -> w479
        tunnel: w478 -> [w502]
        stop <- w501 stop-if-true
        n157 = case shown="True" "Simulation On/Off" {
          tunnel: w506 -> [w508 w527]
          tunnel: w505 -> [w507 w526]
          tunnel: [w510 w525] -> w504
          tunnel: [w509 w524] -> w503
          tunnel: "MtM Z-Axis Input Voltage" -> [_ w523]
          tunnel: "MtM Y-Axis Input Voltage" -> [_ w522]
          tunnel: "MtM X-Axis Input Voltage" -> [_ w521]
          frame False {
            n158 = call-poly <vilib>:"DAQmx Write.vi"("task/channels in"=w508, "data"=dbl[] [0.0, 0.0, 0.0], "error in"=w507) -> ("task out"=w510:refnum<k21>, "error out"=w509:errorcluster)  [unwired: 10 in, 1 out]
            n159 = property on="MtM Y-Axis Input Voltage" class="DigNum (strict)"("DisabledEnum"=T4."Disabled and Grayed Out" ("Disabled"), "Value"=0.0 ("MtM X-Axis Input Voltage")) -> ()  [unwired: 2 in, 2 out]
            n160 = property on="MtM X-Axis Input Voltage" class="DigNum (strict)"("DisabledEnum"=T4."Disabled and Grayed Out" ("Disabled"), "Value"=0.0 ("MtM X-Axis Input Voltage")) -> ()  [unwired: 2 in, 2 out]
            n161 = property on="MtM Z-Axis Input Voltage" class="DigNum (strict)"("DisabledEnum"=T4."Disabled and Grayed Out" ("Disabled"), "Value"=0.0 ("MtM X-Axis Input Voltage")) -> ()  [unwired: 2 in, 2 out]
          }
          frame True {
            n162 = Build Array(w521, w522, w523) -> (w528:dbl[])  [unwired: 1 in]
            n163 = property on="MtM Y-Axis Input Voltage" class="DigNum (strict)"("DisabledEnum"=T4."Enabled" ("Disabled")) -> ()  [unwired: 2 in, 2 out]
            n164 = property on="MtM Z-Axis Input Voltage" class="DigNum (strict)"("DisabledEnum"=T4."Enabled" ("Disabled")) -> ()  [unwired: 2 in, 2 out]
            n165 = property on="MtM X-Axis Input Voltage" class="DigNum (strict)"("DisabledEnum"=T4."Enabled" ("Disabled")) -> ()  [unwired: 2 in, 2 out]
            n166 = call-poly <vilib>:"DAQmx Write.vi"("task/channels in"=w527, "data"=w528, "error in"=w526) -> ("task out"=w525:refnum<k21>, "error out"=w524:errorcluster)  [unwired: 10 in, 1 out]
          }
        }
        n167 = Wait (ms)(milliseconds to wait=u32 100) -> ()  [unwired: 1 out]
        n168 = call <extravilib>:"Read.vi"("channel"=w502) -> ("element"=w501:bool)  [unwired: 1 in, 1 out]
      }
      n169 = call-poly <vilib>:"DAQmx Write.vi"("task/channels in"=w480, "data"=dbl[] [0.0, 0.0, 0.0], "error in"=w479) -> ("task out"=w483:refnum<k21>, "error out"=w482:errorcluster)  [unwired: 10 in, 1 out]
      n170 = call <vilib>:"DAQmx Stop Task.vi"("task/channels in"=w483, "error in"=w482) -> ("task out"=w485:refnum<k21>, "error out"=w484:errorcluster)  [unwired: 12 in]
      n171 = call <vilib>:"DAQmx Clear Task.vi"("task in"=w485, "error in"=w484) -> ()  [unwired: 13 in, 1 out]
    }
    frame Enabled {
    }
  }
  n172 = while {
    tunnel: w43 -> [w553]
    tunnel: w42 -> [w551]
    tunnel: w1 -> [w545]
    stop <- w546 stop-if-true
    n173 = local read "Output 2 Measured Voltage"() -> (w538:string)
    n174 = local read "Output 2 Measured Current"() -> (w539:string)
    n175 = local read "Output 2 Measured Current"() -> (w537:string)
    n176 = local read "Output 1 Measured Voltage"() -> (w544:string)
    n177 = local read "Temperature (Celsius)"() -> (w531:dbl)
    n178 = local read "Output On/Off"() -> (w536:bool)
    n179 = local read "Magnetic Field"() -> (w530:dbl)
    n180 = call <extravilib>:"Read.vi"("channel"=w545) -> ("element"=w546:bool)  [unwired: 1 in, 1 out]
    n181 = Get Date/Time In Seconds() -> (seconds since 1Jan1904=w542:timestamp)
    n182 = shared-variable "NI-PXIe-8880\\Shared Variable Library.lvlib\\X-Axis"() -> (w550:string)  [unwired: 1 in, 1 out]
    n183 = shared-variable "NI-PXIe-8880\\Shared Variable Library.lvlib\\Z-Axis"() -> (w548:string)  [unwired: 1 in, 1 out]
    n184 = shared-variable "NI-PXIe-8880\\Shared Variable Library.lvlib\\Y-Axis"() -> (w549:string)  [unwired: 1 in, 1 out]
    n185 = Get Date/Time String(seconds (now)=w542, want seconds? (F)=TRUE) -> (date string=w541:string, time string=w540:string)  [unwired: 1 in]
    n186 = Boolean To (0,1)(Boolean=w536) -> (0, 1=w535:i16)
    n187 = Number To Fractional String(number=w531) -> (F-format string=w532:string)  [unwired: 3 in]
    n188 = Number To Fractional String(number=w530) -> (F-format string=w533:string)  [unwired: 3 in]
    n189 = Number To Decimal String(number=w535) -> (decimal integer string=w534:string)  [unwired: 1 in]
    n190 = Build Array(w541, w540, w550, w549, w548, w532, w544, w539, w538, w537, w533, w534) -> (w547:string[])
    n191 = call-poly <vilib>:"Write Delimited Spreadsheet.vi"("file path (dialog if empty)"=w553, "1D data"=w547, "append to file? (new file:F)"=TRUE, "error in (no error)"=w551) -> ()  [unwired: 10 in, 2 out]
    n192 = Wait (ms)(milliseconds to wait="Data Record Work Rate (ms)") -> ()  [unwired: 1 out]
  }
  n193 = TCP Close Connection(connection ID=w48, error in (no error)=w47) -> ()  [unwired: 1 in, 2 out]
  n194 = disable-structure shown="Disabled" {
    disable-tunnel: w1 -> [w555 _]
    frame Disabled {
      n195 = TCP Open Connection(address="10.0.194.41", remote port or service name=u16 6444) -> (connection ID=w560:refnum<k5>, error out=w558:errorcluster)  [unwired: 3 in]
      n196 = while {
        tunnel: w560 -> [w573]
        tunnel: [w572] -> w559
        tunnel: w558 -> [w571]
        tunnel: [w570] -> w557
        tunnel: w555 -> [w563]
        stop <- w564 stop-if-true
        n197 = local read "Temperature (Celsius)"() -> (w568:dbl)
        n198 = call <extravilib>:"Read.vi"("channel"=w563) -> ("element"=w564:bool)  [unwired: 1 in, 1 out]
        n199 = shared-variable "NI-PXIe-8880\\Shared Variable Library.lvlib\\X-Axis"() -> (w567:string)  [unwired: 1 in, 1 out]
        n200 = shared-variable "NI-PXIe-8880\\Shared Variable Library.lvlib\\Z-Axis"() -> (w565:string)  [unwired: 1 in, 1 out]
        n201 = shared-variable "NI-PXIe-8880\\Shared Variable Library.lvlib\\Y-Axis"() -> (w566:string)  [unwired: 1 in, 1 out]
        n202 = Format Into String(format string="%s,%s,%s,%f", w567, w566, w565, w568) -> (resulting string=w569:string)  [unwired: 2 in, 1 out]
        n203 = TCP Write(connection ID=w573, data in=w569, error in (no error)=w571, 9:1 ("timeout ms (25000)")) -> (connection ID out=w572:refnum<k5>, error out=w570:errorcluster)  [unwired: 1 out]
      }
      n204 = TCP Close Connection(connection ID=w559, error in (no error)=w557) -> ()  [unwired: 1 in, 2 out]
    }
    frame Enabled {
    }
  }
  n205 = flat-sequence {
    frame #0 {
      n206 = Current VI's Path() -> (path=w575:path)
      n207 = Open VI Reference(vi path=w575) -> (vi reference=w574:refnum<vi>)  [unwired: 5 in, 1 out]
      n208 = invoke class="VI" method="Default Vals.Reinit All"(reference=w574) -> ()  [unwired: 2 in, 3 out]
    }
  }
